vi "format set font name lv.vi"(8 "error in (no error)":errorcluster, 10 "font_name":string, 11 "format":u32) -> (0 "error out":errorcluster)   [LabVIEW 8.6]
doc: "void format_set_font_name_lv(lxw_format format, const char *font_name);"
uses:
  pending_lvxlsxwriter/xlsxwriter.dll
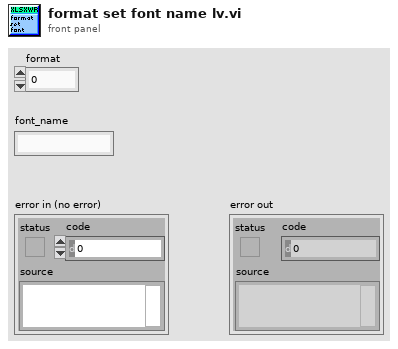
[diagram p1: front panel]
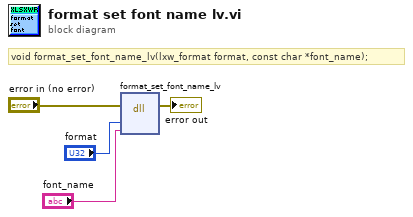
[diagram p0: block diagram]
diagram:
  # "void format_set_font_name_lv(lxw_format format, const char *font_name);"
  n1 = dll-call lib="C:/Users/WDAGUtilityAccount/Desktop/pending_lvxlsxwriter/xlsxwriter.*" fn="format_set_font_name_lv"(error in="error in (no error)", "format"="format", "font_name"="font_name") -> (error out=→"error out":errorcluster)  [unwired: 5 in, 1 out]
